vi "ROI group-Add group to ctrl.vi"(8 "error in (no error)":errorcluster, 11 "Group Name":string) -> (0 "error out":errorcluster)   [LabVIEW 2013]
uses:
  Typedefs/Group sel cluster.ctl
  Global variables/gl_Functional Imaging-Global variables.vi
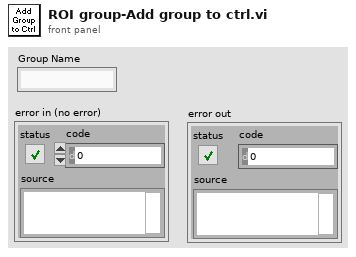
[diagram p1: front panel]
types:
  T1 = typedef "Group sel cluster.ctl" = cluster{"Group number":string, "Group Name":string, "Visibility":bool, "Highlight":bool}
  T2 = typedef "Functional Imging UI Refs.ctl" = cluster{"Menu ref":refnum<k9>, "Image control":refnum<vi>, "VI ref":refnum<vi>, "XGrapher":refnum<vi>, "Smoothing":refnum<vi>, "POI Averaging":refnum<vi>, "Normalize":refnum<vi>, "POI data points in each trial":refnum<vi>, "Channel":refnum<vi>, "Experiment data folder path":refnum<vi>, "[ROI vis]":refnum<vi>, "[Groups] visbl":T3, "Group Name":refnum<vi>, "POI index":refnum<vi>, "Trial No.":refnum<vi>, "Intensity Zoom":refnum<vi>, "Trial Cursor Enabled":refnum<vi>, "Number of Trials (ind 1)":refnum<vi>, "Number of Trials (ind 2)":refnum<vi>, "MiniScans Available":refnum<vi>, "POI Available":refnum<vi>, "Defer graph updates":refnum<vi>, "Waveform selector":refnum<vi>, "#of selected POI":refnum<vi>, "#of selected MiniScans":refnum<vi>, "#of selected groups":refnum<vi>, "Max Z-Projection":refnum<vi>, "Z-Plane Selector":refnum<vi>, "Index of miniscan point to visualise":refnum<vi>, "ROI vis. mode":refnum<vi>, "Total # of points":refnum<vi>, "Index of group clicked on":refnum<vi>, "Pane 1":refnum<vi>, "Pane 2":refnum<vi>, "Pane 3":refnum<vi>, "Pane 4":refnum<vi>, "Pane 5":refnum<vi>, "Pane 6":refnum<vi>, "Deselect all ROI":refnum<vi>, "Deselect all groups":refnum<vi>}
  T3 = typedef "Groups array referecne.ctl" = refnum<vi>
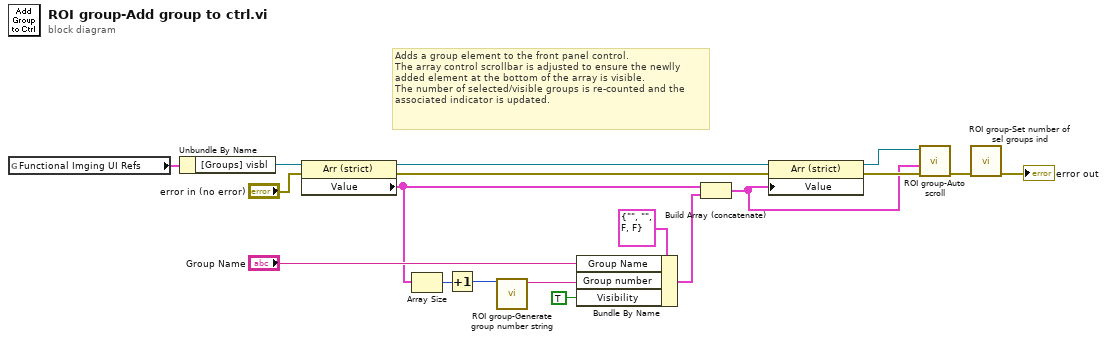
[diagram p0: block diagram]
diagram:
  # "Adds a group element to the front panel control.\nThe array control scrollbar is adjusted to ensure the newlly added element at the bottom of the array is visible.\nThe number of selected/visible groups is re-counted and the associated indicator is updated."
  n1 = global read "gl_Functional Imaging-Global variables.vi" "Functional Imging UI Refs"() -> (w3:T2)
  n2 = Unbundle By Name(w3) -> ("[Groups] visbl"=w7:T3)
  n3 = property on="Property Node" class="Arr (strict)"(reference=w7, error in="error in (no error)") -> (reference out=w18:T3, error out=w16:errorcluster, "Value"=w5:T1[])
  n4 = Array Size(array=w5) -> (size(s)=w4:i32)
  n5 = Increment(x=w4) -> (x+1=w2:i32)
  n6 = call "ROI group-Generate group number string.vi"("Group number"=w2) -> ("Group number string"=w1:string)  [unwired: 10 in]
  n7 = Bundle By Name(cluster=T1 {"Group number"="", "Group Name"="", "Visibility"=FALSE, "Highlight"=FALSE} ("POI sel & vis"), "Group Name"="Group Name", "Group number"=w1, "Visibility"=TRUE) -> (w14:T1)
  n8 = Build Array (concatenate)(w5, w14) -> (w6:T1[])
  n9 = property on="Property Node" class="Arr (strict)"(reference=w18, error in=w16, "Value"=w6) -> (reference out=w10:T3, error out=w9:errorcluster)
  n10 = call "ROI group-Auto scroll.vi"("error in (no error)"=w9, "Array"=w6, "[Groups]"=w10) -> ("error out"=w8:errorcluster)  [unwired: 8 in]
  n11 = call "ROI group-Set number of sel groups ind.vi"("error in (no error)"=w8) -> ("error out"=→"error out":errorcluster)  [unwired: 10 in]
